vi "AVI-Time series subset export-setup.vi"(11 "AVI path & name":path) -> (0 "error out":errorcluster, 1 "AVI modes refs":T2, 2 "AVI Refnum (duplicate)":T1, 3 "# of Frames in exported portion":i32, 4 "Extraction cursors":cluster{"Min cursor":i32, "Max cursor":i32}, 5 "Export all split AVI files as one":bool)   [LabVIEW 2020]
uses:
  Typedefs/AVI modes refs cluster.ctl
  <vilib>/vision/Avi1.llb/AviRefnum.ctl
  <vilib>/vision/Avi.llb/IMAQ AVI2 Refnum.ctl
  Globals/gl_Time series viewer globals.vi
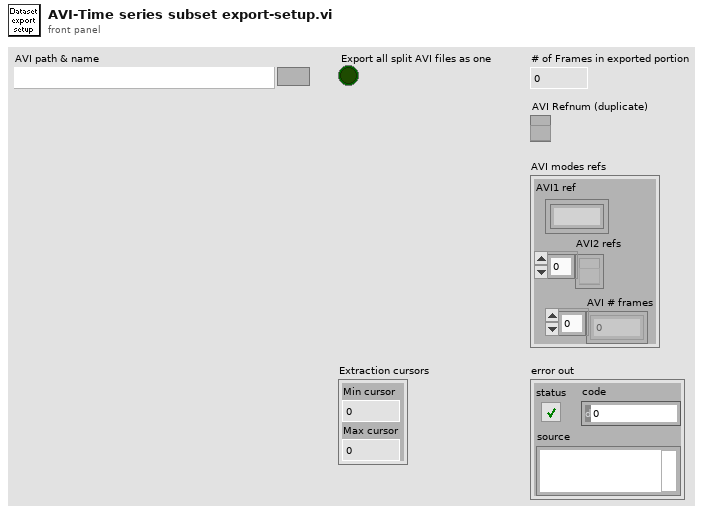
[diagram p1: front panel]
types:
  T1 = typedef "IMAQ AVI2 Refnum.ctl" = refnum<k20>
  T2 = typedef "AVI modes refs cluster.ctl" = cluster{"AVI1 ref":T3, "AVI2 refs":T1[], "AVI # frames":u32[]}
  T3 = typedef "AviRefnum.ctl" = refnum<k1>
  T4 = typedef "Time series viewer refs.ctl" = cluster{"This VI":refnum<vi>, "Image control":refnum<vi>, "AVI Mode ind":refnum<vi>, "Play":refnum<vi>, "Stop":refnum<vi>, "Back":refnum<vi>, "Scrollbar":refnum<vi>, "Video length info":refnum<vi>, "Expected speed values":refnum<vi>, "Intensity":refnum<vi>, "Path":refnum<vi>, "Selection sliders":refnum<vi>, "Speed Graph ref":refnum<vi>, "Frame rate set (fps)":refnum<vi>, "Number of rows to generate":refnum<vi>, "VL Image Array":refnum<vi>, "Image Scrollbar":refnum<vi>, "Channel to load":refnum<vi>, "Colour":refnum<vi>}
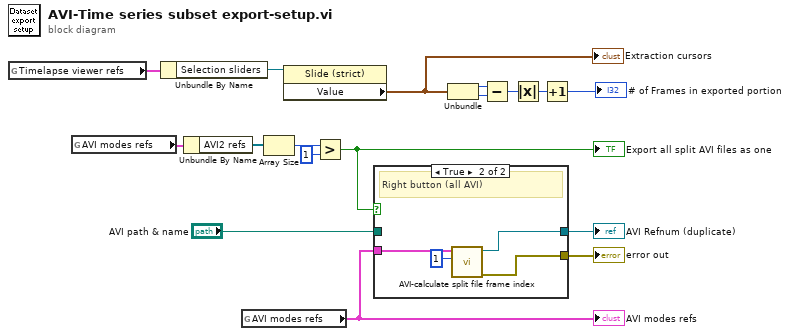
[diagram p0: block diagram]
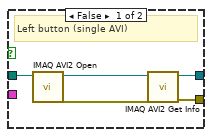
[diagram p2: hidden frame]
diagram:
  n1 = global read "gl_Time series viewer globals.vi" "Timelapse viewer refs"() -> (w8:T4)
  n2 = global read "gl_Time series viewer globals.vi" "AVI modes refs"() -> (w16:T2)
  n3 = Unbundle By Name(w8) -> ("Selection sliders"=w9:refnum<vi>)
  n4 = Unbundle By Name(w16) -> ("AVI2 refs"=w15:T1[])
  n5 = global read "gl_Time series viewer globals.vi" "AVI modes refs"() -> (w11:T2)
  "AVI modes refs" <- w11
  n6 = Array Size(array=w15) -> (size(s)=w14:i32)
  n7 = property class="Slide (strict)"(reference=w9) -> ("Value"=w2:cluster{i32, i32})  [unwired: 1 in, 2 out]
  "Extraction cursors" <- w2
  n8 = Greater?(x=w14, y=1) -> (0:w10:bool)
  "Export all split AVI files as one" <- w10
  n9 = case shown="True" w10 {
    tunnel: "AVI path & name" -> [w20 _]
    tunnel: [w19 w25] -> w12
    tunnel: w11 -> [_ w26]
    tunnel: [w18 w23] -> w1
    frame False {
      # "Left button (single AVI)"
      n10 = call "IMAQ AVI2 Open"("AVI File Path"=w20) -> ("error out"=w22:errorcluster, "AVI Refnum"=w21:T1)  [unwired: 9 in]
      n11 = call "IMAQ AVI2 Get Info"("error in (no error)"=w22, "AVI Refnum"=w21) -> ("error out"=w18:errorcluster, "AVI Refnum (duplicate)"=w19:T1)  [unwired: 5 in, 3 out]
    }
    frame True {
      # "Right button (all AVI)"
      n12 = call "AVI-calculate split file frame index.vi"("Frame number (unity-based) in"=1, "AVI modes refs"=w26) -> ("error out"=w23:errorcluster, "AVI2 split file ref"=w25:T1)  [unwired: 6 in, 2 out]
    }
  }
  "AVI Refnum (duplicate)" <- w12
  "error out" <- w1
  n13 = Unbundle(w2) -> (w7:i32, w6:i32)
  n14 = Subtract(x=w7, y=w6) -> (x-y=w5:i32)
  n15 = Absolute Value(x=w5) -> (abs(x)=w4:i32)
  n16 = Increment(x=w4) -> (x+1=→"# of Frames in exported portion":i32)
